vi "NISE.remote.Property Node Write Core.vi"(8 "error in (no error)":errorcluster, 9 "JSON Value in":refnum<class "JSON Value.lvclass">, 10 "property":string, 11 "SLSC Remote in":refnum<class "SLSC Interface.lvclass">) -> (0 "error out":errorcluster, 3 "SLSC Remote out":refnum<class "SLSC Interface.lvclass">)   [LabVIEW 2016, in "SLSC Interface.lvclass"]
uses:
  SLSC Interface Class/SLSC Interface.lvclass
  <vilib>/NI/JSON Support for LabVIEW/JSON Value/JSON Value.lvclass
  SLSC Interface Class/SLSC Interface.lvclass/SLSC Interface.ctl
  SLSC Interface Class/NISE.Read client handle.vi
  SLSC Interface Class/NISE.Read URL.vi
  SLSC Interface Class/NISE.Read session.vi
  <vilib>/httpClient/POSTBuffer.vi
  <vilib>/httpClient/LabVIEWHTTPClient.lvlib
  <vilib>/NI/NI JSONRPC Server Framework/Classes/Client/JSONRPC Client.lvclass
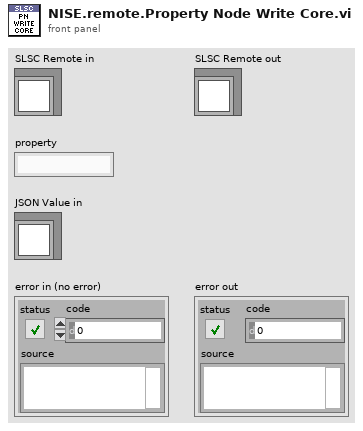
[diagram p1: front panel]
types:
  T1 = typedef "LabVIEWHTTPClient.lvlib/ClientHandle.ctl" = refnum<k1>
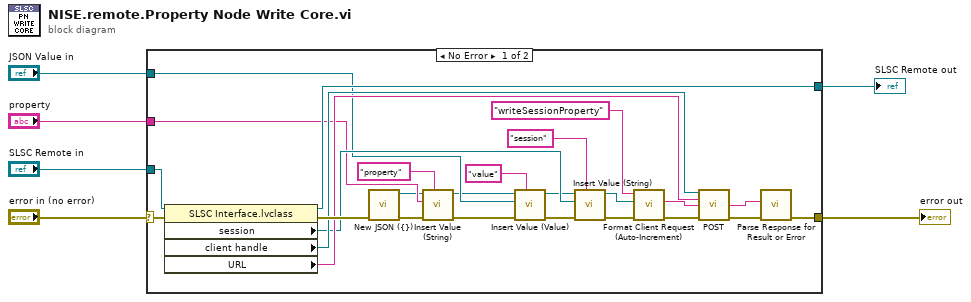
[diagram p0: block diagram]
diagram:
  n1 = case shown="No Error" "error in (no error)" {
    selector: "error in (no error)" -> [w30 w33]
    tunnel: "SLSC Remote in" -> [w32 w34]
    tunnel: [w31 w34] -> w3
    tunnel: [w18 w33] -> w4
    tunnel: "property" -> [w10 _]
    tunnel: "JSON Value in" -> [w11 _]
    frame No Error {
      n2 = property class="SLSC Interface.lvclass"(reference=w32, error in=w30) -> (reference out=w31:refnum<class "SLSC Interface.lvclass">, error out=w29:errorcluster, "session"=w12:refnum<k21>, "client handle"=w23:T1, "URL"=w22:string)
      n3 = call <vilib>:"New JSON ({}).vi"("error in (no error)"=w29) -> ("error out"=w28:errorcluster, "JSON Value out"=w9:refnum<class "JSON Value.lvclass">)  [unwired: 9 in]
      n4 = call <vilib>:"Insert Value (String).vi"("key"="property" ("Name"), "error in (no error)"=w28, "value"=w10, "JSON Value in"=w9) -> ("error out"=w16:errorcluster, "JSON Value out"=w8:refnum<class "JSON Value.lvclass">)  [unwired: 5 in, 1 out]
      n5 = call <vilib>:"Insert Value (Value).vi"("key"="value" ("Name"), "error in (no error)"=w16, 10:"JSON Value in"=w11, 11:"JSON Value in"=w8) -> ("error out"=w17:errorcluster, "JSON Value out"=w7:refnum<class "JSON Value.lvclass">)  [unwired: 5 in, 1 out]
      n6 = call <vilib>:"Insert Value (String).vi"("key"="session" ("Name"), "error in (no error)"=w17, "value"=w12, "JSON Value in"=w7) -> ("error out"=w24:errorcluster, "JSON Value out"=w25:refnum<class "JSON Value.lvclass">)  [unwired: 5 in, 1 out]
      n7 = call <vilib>:"Format Client Request (Auto-Increment).vi"("error in (no error)"=w24, "JSON Value in"=w25, "method"="writeSessionProperty") -> ("error out"=w21:errorcluster, "Request String"=w26:string)  [unwired: 7 in]
      n8 = call-poly <vilib>:"POST.vi"("client handle"=w23, "url"=w22, "buffer"=w26, "error in (no error)"=w21) -> ("body"=w20:string, "error out"=w19:errorcluster)  [unwired: 8 in, 2 out]
      n9 = call <vilib>:"Parse Response for Result or Error.vi"("error in"=w19, "Response String In"=w20) -> ("error out"=w18:errorcluster)  [unwired: 7 in, 2 out]
    }
    frame Error {
    }
  }
  "error out" <- w4
  "SLSC Remote out" <- w3
